vi "ROI.vi"() -> ()   [LabVIEW 2014]
doc: "This example gets you started with ROI operations.\n\nFor convenient ROI selection we use the IMAQ Image control. \nIt is also possible to programmatically set the ROI properties and work without IMAQ / NI Vision."
uses:
  MSC Image_class/controls/Image Type.ctl
  MSC Image_class/MSC Image.lvclass
panel:
  out "Tree":string(tree)
  in  "stop":bool
  out "IMAQ Image":T1(plugin-control)
  out "error out":errorcluster
  out "Extracted ROI":picture
  # "Select multiple ROIs with Ctrl-Click"
  # "Results are displayed here"
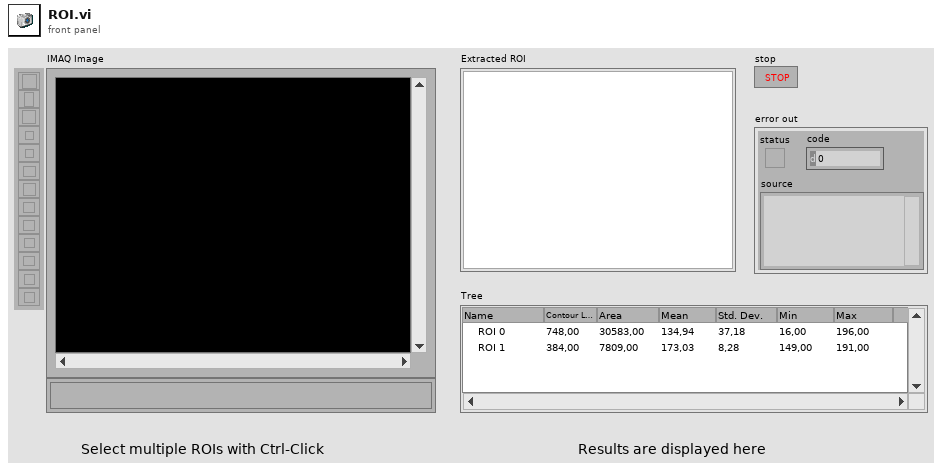
[diagram p1: front panel]
types:
  T1 = typedef "IMAQ Image.ctl" = refnum<image>
  T2 = cluster{"Global Rectangle":i32[], "Contours":cluster{"Contour Type":u32, "ROI Type":u32, "Points":i32[]}[]}
  T3 = typedef "MSC Image.lvclass/Image Type.ctl" = i32
  T4 = typedef "MSC Image.lvclass/ROI.ctl" = cluster{"Type":T5, "Parameters":dbl[], "Contour":T6, "Bounding Box":T6, "Contour Length":dbl, "ROI Area":dbl, "ROI Mean":dbl, "ROI Standard Deviation":dbl, "ROI Min":dbl, "ROI Max":dbl, "Hierarchy":T7, "Variant":variant, "Timestamp":timestamp}
  T5 = typedef "MSC Image.lvclass/ROI Type.ctl" = u16
  T6 = typedef "MSC Image.lvclass/Contour.ctl" = cluster{"x":i16, "y":i16}[]
  T7 = typedef "MSC Image.lvclass/Contour hierarchy.ctl" = cluster{"parent ID":i32, "children IDs":dbl[], "level":i32}
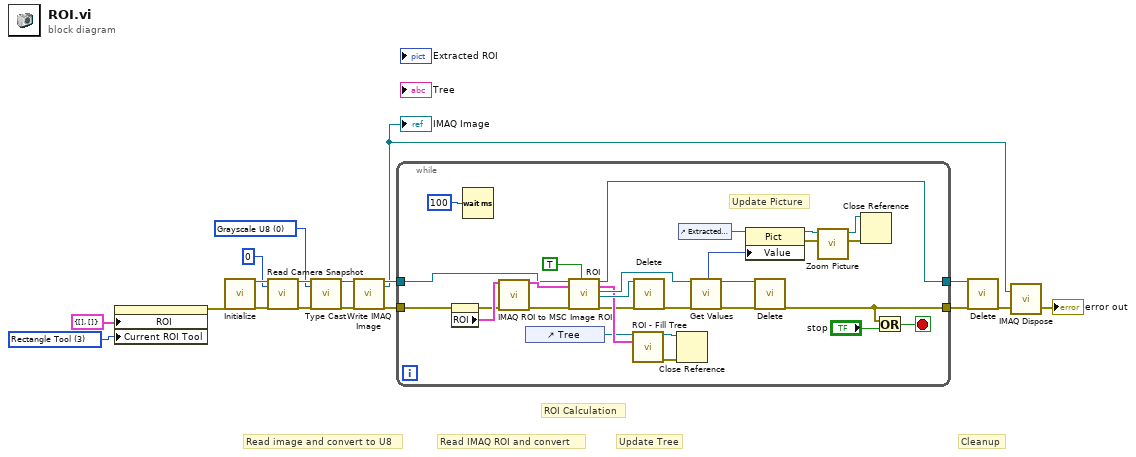
[diagram p0: block diagram]
diagram:
  w3 = u32 3 items=["Zoom Tool"=8, "Selection Tool"=0, "Pan Tool"=9, "Point Tool"=1, "Line Tool"=2, "Rectangle Tool"=3, "Rotated Rectangle Tool"=12, "Polyline Tool"=10, "Polygon Tool"=5, "Freehand Tool"=11, "Closed Freehand Tool"=6, "Ellipse Tool"=4, "Annulus Tool"=7] ("Current ROI Tool")
  w9 = T3 0 items=["Grayscale U8"=0, "Grayscale U16"=2, "Grayscale Single"=5, "Grayscale Double"=6, "RGB U8"=16] ("Image Type")
  # "Update Tree"
  # "ROI Calculation"
  # "Read IMAQ ROI and convert"
  # "Cleanup"
  # "Read image and convert to U8"
  n1 = property on="IMAQ Image" class="ImageControl"("ROI"=T2 {"Global Rectangle"=[], "Contours"=[]}, "Current ROI Tool"=w3) -> (error out=w5:errorcluster)  [unwired: 2 in, 1 out]
  n2 = call "Initialize.vi"("error in (no error)"=w5) -> ("image out"=w18:refnum<class "MSC Image.lvclass">, "error out"=w17:errorcluster)  [unwired: 17 in]
  n3 = call-dynamic "Read Camera Snapshot.vi"("image in"=w18, "camID"=0, "error in (no error)"=w17) -> ("image out"=w15:refnum<class "MSC Image.lvclass">, "error out"=w8:errorcluster)  [unwired: 15 in]
  n4 = call-dynamic "Type Cast.vi"("image in"=w15, "Image Type"=w9, "error in (no error)"=w8) -> ("image out"=w2:refnum<class "MSC Image.lvclass">, "error out"=w1:errorcluster)  [unwired: 15 in]
  n5 = call-dynamic "Write IMAQ Image.vi"("image in"=w2, "error in (no error)"=w1) -> ("image out"=w14:refnum<class "MSC Image.lvclass">, "IMAQ Image out"=w13:T1, "error out"=w7:errorcluster)  [unwired: 15 in]
  "IMAQ Image" <- w13
  n6 = while {
    tunnel: w14 -> [w44]
    tunnel: [w43] -> w12
    tunnel: w7 -> [w26]
    tunnel: [w21] -> w6
    stop <- w19 stop-if-true
    # "Update Picture"
    n7 = property on="IMAQ Image" class="ImageControl"(error in=w26) -> (error out=w23:errorcluster, "ROI"=w46:T2)  [unwired: 1 in, 1 out]
    n8 = Wait (ms)(milliseconds to wait=u32 100) -> ()  [unwired: 1 out]
    n9 = call "IMAQ ROI to MSC Image ROI.vi"("IMAQ ROI Descriptor"=w46, "error in"=w23) -> ("ROIs"=w45:T4[], "error out"=w22:errorcluster)  [unwired: 12 in]
    n10 = control-ref of="Tree"() -> (w31:refnum<vi>)
    n11 = call-dynamic "ROI.vi"("image in"=w44, "ROIs In"=w45, "error in (no error)"=w22, "Crop?"=TRUE) -> ("image out"=w43:refnum<class "MSC Image.lvclass">, "ROIs Out"=w38:T4[], "particle image out"=w41:refnum<class "MSC Image.lvclass">, "particle mask image out"=w42:refnum<class "MSC Image.lvclass">, "error out"=w27:errorcluster)  [unwired: 11 in]
    n12 = call "ROI - Fill Tree.vi"("TreeControl in"=w31, "ROIs"=w38) -> ("TreeControl out"=w30:refnum<vi>, "error out"=w29:errorcluster)  [unwired: 11 in, 1 out]
    n13 = call-dynamic "Delete.vi"("image in"=w42, "error in (no error)"=w27) -> ("error out"=w28:errorcluster)  [unwired: 17 in]
    n14 = Close Reference(reference=w30, error in (no error)=w29) -> ()  [unwired: 1 out]
    n15 = control-ref of="Extracted ROI"() -> (w37:refnum<vi>)
    n16 = call-dynamic "Get Values.vi"("image in"=w41, "error in (no error)"=w28) -> ("picture"=w36:picture, "image out"=w40:refnum<class "MSC Image.lvclass">, "error out"=w39:errorcluster)  [unwired: 10 in, 5 out]
    n17 = property class="Pict"(reference=w37, "Value"=w36) -> (reference out=w35:refnum<vi>, error out=w34:errorcluster)  [unwired: 1 in]
    n18 = call-dynamic "Delete.vi"("image in"=w40, "error in (no error)"=w39) -> ("error out"=w21:errorcluster)  [unwired: 17 in]
    n19 = call "Zoom Picture.vi"("error in (no error)"=w34, "Picture in"=w35) -> ("error out"=w32:errorcluster, "Picture out"=w33:refnum<vi>)  [unwired: 8 in]
    n20 = Close Reference(reference=w33, error in (no error)=w32) -> ()  [unwired: 1 out]
    n21 = Or(x=w21, y="stop") -> (x .or. y?=w19:bool)
  }
  n22 = call-dynamic "Delete.vi"("image in"=w12, "error in (no error)"=w6) -> ("error out"=w11:errorcluster)  [unwired: 17 in]
  n23 = call "IMAQ Dispose"("Image"=w13, "error in (no error)"=w11) -> ("error out"=→"error out":errorcluster)  [unwired: 4 in]
